vi "Get Shooter Info.vi"(11 "Dashboard Packet":T1) -> (1 "Right Wheel Target":dbl, 2 "Left Wheel Target":dbl, 3 "Target Angle":dbl)   [LabVIEW 2016]
uses:
  Common Code/Dashboard Control Data.ctl
  Common Code/Drivetrain Settings.ctl
  Common Code/Intake Presets.ctl
  Common Code/Shooter Presets.ctl
  Robot Global Data.vi
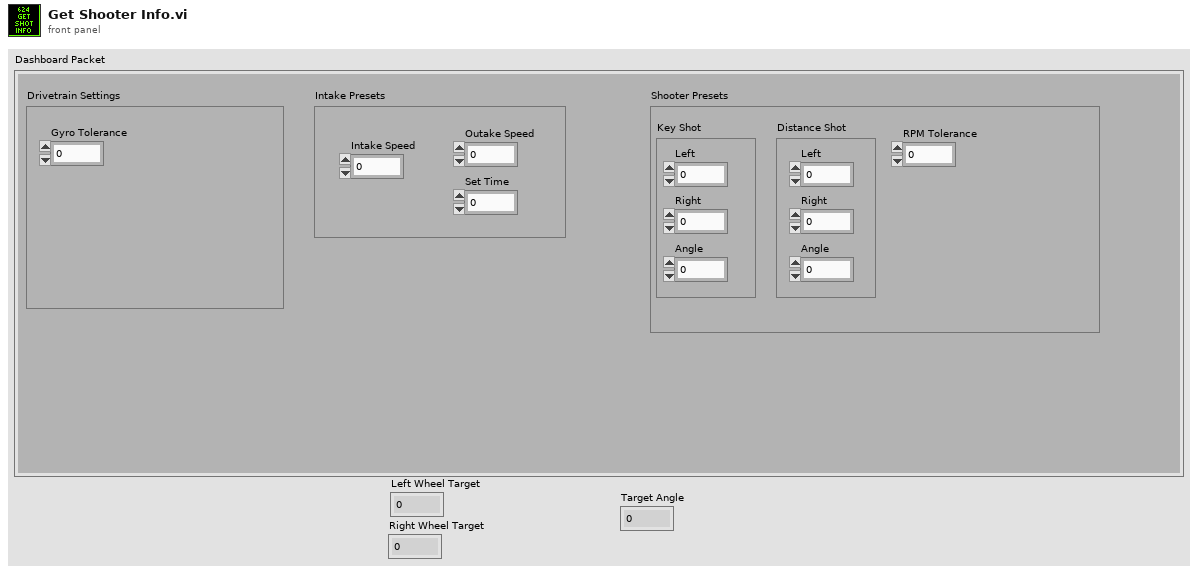
[diagram p1: front panel]
types:
  T1 = typedef "Dashboard Control Data.ctl" = cluster{"Drivetrain Settings":T2, "Intake Presets ":T3, "Shooter Presets":T4}
  T2 = typedef "Drivetrain Settings.ctl" = cluster{"Gyro Tolerance":dbl}
  T3 = typedef "Intake Presets.ctl" = cluster{"Intake Speed ":dbl, "Outake Speed":dbl, "Set Time":dbl}
  T4 = typedef "Shooter Presets.ctl" = cluster{"Key Shot":cluster{"Left ":dbl, "Right":dbl, "Angle":dbl}, "Distance Shot":cluster{"Left":dbl, "Right":dbl, "Angle":dbl}, "RPM Tolerance":dbl}
  T5 = typedef "Shooter Command Cluster.ctl" = cluster{"Y Power":dbl, "Modes":T6, "Shot Types":T7, "Auto Commands":T8}
  T6 = typedef "Shooter Modes.ctl" = enum16{"Manual", "Auto"}
  T7 = typedef "Shot Types.ctl" = enum16{"Key", "Distance"}
  T8 = typedef "Auto Shoot Commands.ctl" = enum16{"Idle", "Warmup", "Shoot"}
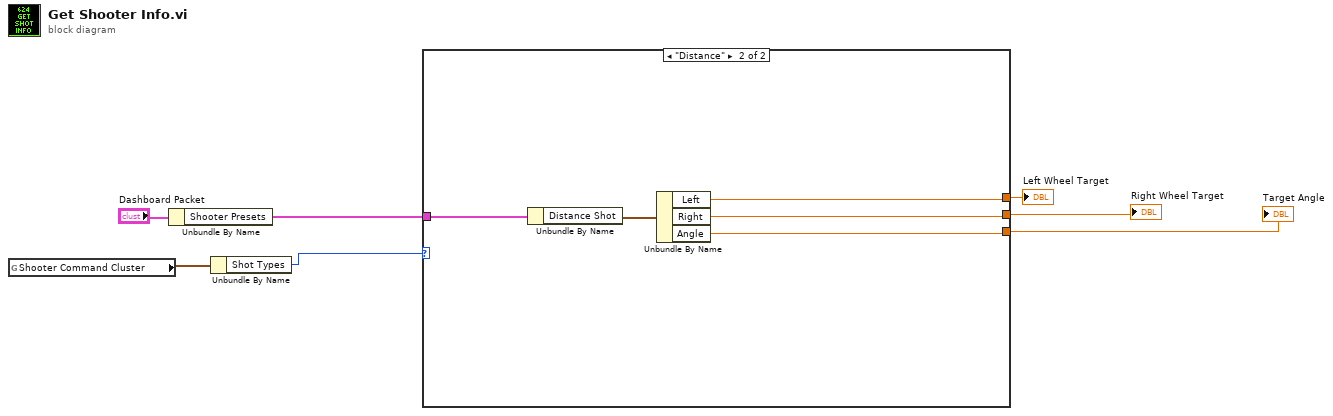
[diagram p0: block diagram]
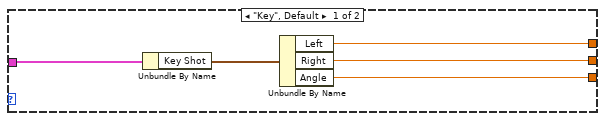
[diagram p2: hidden frame]
diagram:
  n1 = global read "Robot Global Data.vi" "Shooter Command Cluster"() -> (w6:T5)
  n2 = Unbundle By Name("Dashboard Packet") -> ("Shooter Presets"=w4:T4)
  n3 = Unbundle By Name(w6) -> ("Shot Types"=w5:T7)
  n4 = case shown="\"Distance\"" w5 {
    tunnel: w4 -> [w12 w17]
    tunnel: [w10 w15] -> w3
    tunnel: [w9 w14] -> w2
    tunnel: [w8 w13] -> w1
    frame "Key", Default {
      n5 = Unbundle By Name(w12) -> ("Key Shot"=w11:cluster{"Left ":dbl, "Right":dbl, "Angle":dbl})
      n6 = Unbundle By Name(w11) -> ("Left"=w10:dbl, "Right"=w9:dbl, "Angle"=w8:dbl)
    }
    frame "Distance" {
      n7 = Unbundle By Name(w17) -> ("Distance Shot"=w16:cluster{"Left":dbl, "Right":dbl, "Angle":dbl})
      n8 = Unbundle By Name(w16) -> ("Left"=w15:dbl, "Right"=w14:dbl, "Angle"=w13:dbl)
    }
  }
  "Left Wheel Target" <- w3
  "Right Wheel Target" <- w2
  "Target Angle" <- w1
